vi "Set Output.vi"(0 "COM Port":string="COM3", 5 "Primary Voltage":dbl, 7 "Delay Time (s)":dbl, 9 "Output Type":i32(ring) items=["DC Volts", "AC Volts", "DC Current", "AC Current", "DC Power", "AC Power", "Dual DC Volts", "Dual AC Volts", "Resistance"], 11 "error in":errorcluster, 12 "Output Enabled":bool) -> (15 "error out":errorcluster)   [LabVIEW 2015]
uses:
  <instrlib>/Fluke 5080/Fluke 5080.lvlib
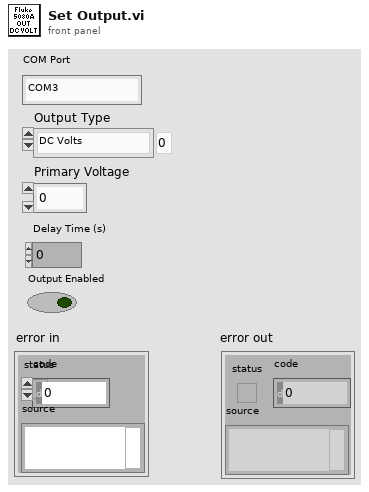
[diagram p1: front panel]
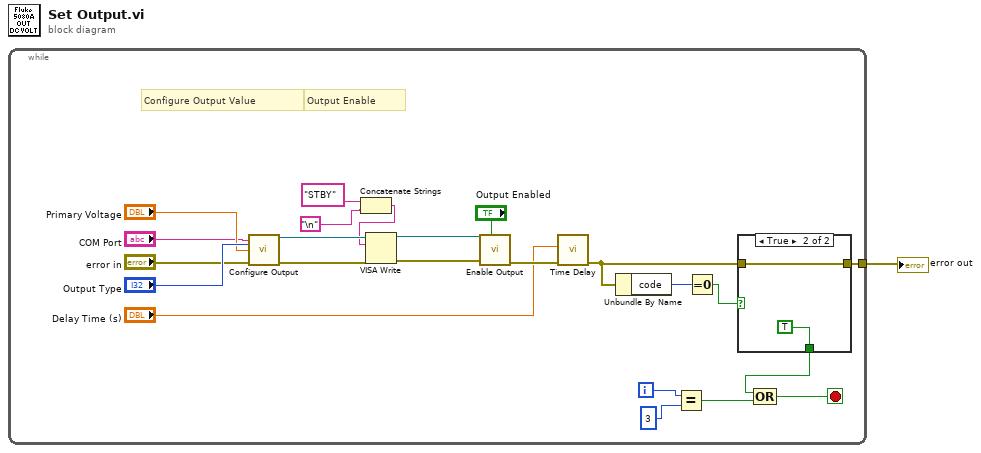
[diagram p0: block diagram]
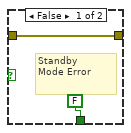
[diagram p2: hidden frame]
diagram:
  n1 = while {
    tunnel: [w10] -> w1
    i -> [w15]
    stop <- w12 stop-if-true
    # "Output Enable"
    # "Configure Output Value"
    n2 = call <instrlib>:"Configure Output.vi"("VISA resource name"="COM Port", "Output Type (0: DC Volts)"="Output Type", "Primary Voltage (5.0)"="Primary Voltage", "error in (no error)"="error in") -> ("VISA resource name out"=w6:refnum<visa-resource-name>, "error out"=w5:errorcluster)  [unwired: 6 in, 4 out]
    n3 = Concatenate Strings("STBY" ("write buffer"), "\n") -> (w2:string)
    n4 = VISA Write(VISA resource name=w6, write buffer=w2, error in (no error)=w5) -> (VISA resource name out=w20:refnum<visa-resource-name>, error out=w19:errorcluster)  [unwired: 1 out]
    n5 = call <instrlib>:"Enable Output.vi"("Output Enabled (T: Enable)"="Output Enabled", "error in (no error)"=w19, "VISA resource name"=w20) -> ("error out"=w21:errorcluster)  [unwired: 8 out]
    n6 = call "Time Delay"("error in (no error)"=w21, "Delay Time (s)"="Delay Time (s)") -> ("error out"=w11:errorcluster)  [unwired: 9 in]
    n7 = Unbundle By Name(w11) -> ("code"=w18:i32)
    n8 = Equal?(x=w15, y=3) -> (x = y?=w13:bool)
    n9 = Equal To 0?(x=w18) -> (x = 0?=w17:bool)
    n10 = case shown="True" w17 {
      tunnel: [FALSE TRUE] -> w14
      tunnel: w11 -> [w25 w27]
      tunnel: [w25 w27] -> w10
      frame False {
        # "Standby\nMode Error"
      }
      frame True {
      }
    }
    n11 = Compound Arithmetic op=OR(w14, w13) -> (w12:bool)
  }
  "error out" <- w1
